vi "TemplateLoadUI.vi"(11 "BasePath":path) -> (2 "Cancelled?":bool, 3 "Steps":T1(array[cluster]))   [LabVIEW 2016]
uses:
  <vilib>/Utility/file.llb/Read Delimited Spreadsheet (string).vi
panel:
  out "AscriptLines":string[](array[string])
  in  "Autoscript Layout":string(tree)
  in  "Arguments":T2
  in  "TemplateFiles":i32(listbox)=7
  in  "Cancel Button":bool
  in  "Add Button":bool
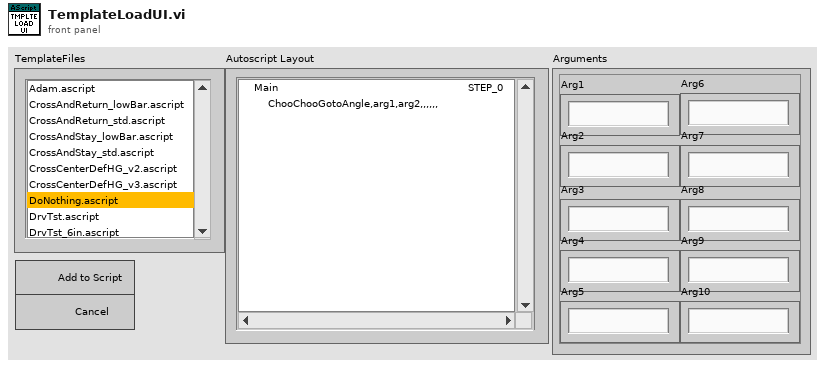
[diagram p1: front panel]
types:
  T1 = cluster{"Number":i32, "Name":string, "Commands":string[], "WaitForExecution":bool}[]
  T2 = cluster{"Arg1":string, "Arg2":string, "Arg3":string, "Arg4":string, "Arg5":string, "Arg6":string, "Arg7":string, "Arg8":string, "Arg9":string, "Arg10":string}
  T3 = cluster{"Number":i32, "Name":string, "Commands":string[], "WaitForExecution":bool}
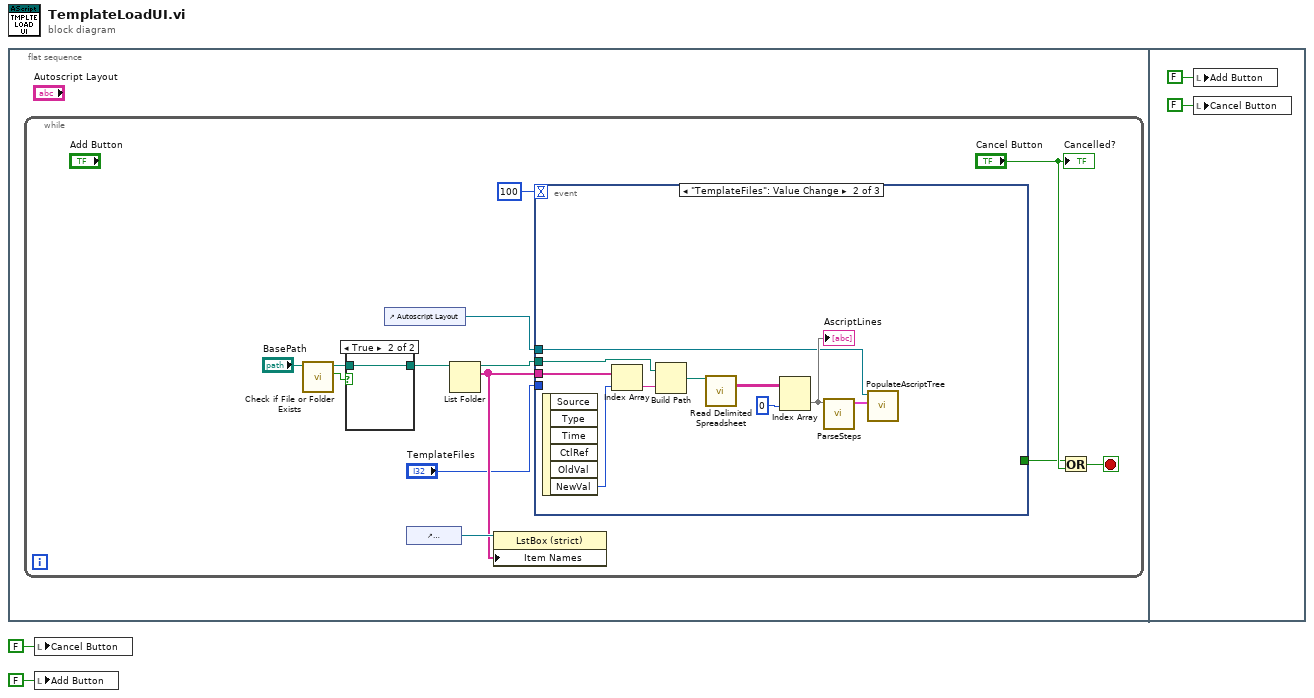
[diagram p0: block diagram]
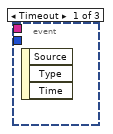
[diagram p2: hidden frame]
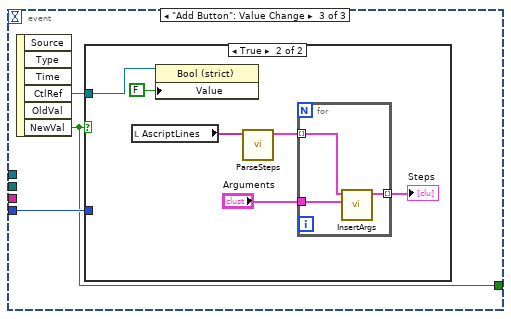
[diagram p3: hidden frame]
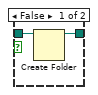
[diagram p5: hidden frame]
diagram:
  n1 = flat-sequence {
    frame #0 {
      n2 = while {
        stop <- w5 stop-if-true
        n3 = call <vilib>:"Check if File or Folder Exists.vi"("path"="BasePath") -> ("file or folder exists?"=w15:bool, "dup path"=w14:path)  [unwired: 8 in, 1 out]
        n4 = case shown="True" w15 {
          tunnel: w14 -> [w39 w40]
          tunnel: [w38 w40] -> w13
          frame False {
            n5 = Create Folder(path (use dialog)=w39) -> (created path=w38:path)  [unwired: 2 in, 2 out]
          }
          frame True {
          }
        }
        n6 = control-ref of="Autoscript Layout"() -> (w4:refnum<vi>)
        n7 = control-ref of="TemplateFiles"() -> (w12:refnum<vi>)
        n8 = List Folder(path=w13) -> (path out=w9:path, filenames=w11:string[])  [unwired: 3 in, 2 out]
        n9 = property on="Property Node" class="LstBox (strict)"(reference=w12, "Item Names"=w11) -> ()  [unwired: 1 in, 2 out]
        n10 = event shown="[1] \"TemplateFiles\": Value Change" {
          selector: _ -> [_ _ _]
          dyn-events: _ -> [_ _ _]
          timeout: 100 -> [_ _ _]
          tunnel: w11 -> [_ w24 _]
          tunnel: w9 -> [_ w22 _]
          tunnel: "TemplateFiles" -> [_ _ w28]
          tunnel: [_ _ w26] -> w6
          tunnel: w4 -> [_ w16 _]
          event Timeout {
            n11 = event-data() -> ()  [unwired: 1 in, 3 out]
          }
          event "TemplateFiles": Value Change {
            n12 = event-data() -> ("NewVal"=w25:i32)  [unwired: 1 in, 5 out]
            n13 = Index Array(array=w24, index=w25) -> (element=w23:string)
            n14 = Build Path(base path=w22, name or relative path=w23) -> (appended path=w19:path)
            n15 = call-poly <vilib>:"Read Delimited Spreadsheet.vi"("file path (dialog if empty)"=w19) -> ("all rows"=w20:string[][])  [unwired: 9 in, 5 out]
            n16 = Index Array(array=w20, index (col)=0 ("disabled index (col)")) -> (element=w18:string[])  [unwired: 1 in]
            "AscriptLines" <- w18
            n17 = call "ParseSteps.vi"("AscriptLines"=w18) -> ("Steps"=w17:T1)  [unwired: 10 in]
            n18 = call "PopulateAscriptTree.vi"("Steps in"=w17, "Autoscript Layout"=w16) -> ()  [unwired: 8 in, 2 out]
          }
          event "Add Button": Value Change {
            n19 = event-data() -> ("CtlRef"=w27:refnum<vi>, "NewVal"=w26:bool)  [unwired: 1 in, 4 out]
            n20 = case shown="True" w26 {
              tunnel: w28 -> [_ _]
              tunnel: w27 -> [_ w34]
              frame False {
              }
              frame True {
                n21 = local read "AscriptLines"() -> (w32:string[])
                n22 = property class="Bool (strict)"(reference=w34, "Value"=FALSE) -> ()  [unwired: 1 in, 2 out]
                n23 = call "ParseSteps.vi"("AscriptLines"=w32) -> ("Steps"=w31:T1)  [unwired: 10 in]
                n24 = for {
                  tunnel: w31 -> [w37] mode=indexing
                  tunnel: "Arguments" -> [w36]
                  tunnel: [w35] -> w29 mode=indexing
                  n25 = call "InsertArgs.vi"("Arguments"=w36, "StepIn"=w37) -> ("StepOut"=w35:T3)  [unwired: 9 in]
                }
                "Steps" <- w29
              }
            }
          }
        }
        n26 = Or(x=w6, y="Cancel Button") -> (x .or. y?=w5:bool)
        "Cancelled?" <- "Cancel Button"
      }
    }
    frame #1 {
      n27 = local write "Add Button"(FALSE ("Cancel Button")) -> ()
      n28 = local write "Cancel Button"(FALSE ("Cancel Button")) -> ()
    }
  }
  n29 = local write "Cancel Button"(FALSE ("Cancel Button")) -> ()
  n30 = local write "Add Button"(FALSE ("Cancel Button")) -> ()
